vi "LV8_10a.vi"() -> ()   [LabVIEW 2016]
uses:
  <vilib>/imath/engines/lvmath2/RunTimeEngine/RangeToken/NIMS_Range.vi
  <instcachedir>/0/NIMS_Range_A7C094595B484CA7AF10685B02D808ED.lvgen/NIMS_Range_A7C094595B484CA7AF10685B02D808ED_000.vi
  <vilib>/imathl/engines/lvmath/Functions/Error Handling/Create Error.vi
  <vilib>/imath/engines/lvmath2/RunTimeEngine/BuiltInFunctions/abs/NIMS_abs(signed).vi
  <instcachedir>/0/NIMS_abs(signed)_C4FCB8E6058B49B797C7C8D53CA5F6EC.lvgen/NIMS_abs(signed)_C4FCB8E6058B49B797C7C8D53CA5F6EC_001.vi
  <vilib>/imath/engines/lvmath2/RunTimeEngine/BuiltInFunctions/fft/NIMS_fft(GV).vi
  <instcachedir>/0/NIMS_fft(GV)_4C6467FC22F84E4BA42517A07EF978B0.lvgen/NIMS_fft(GV)_4C6467FC22F84E4BA42517A07EF978B0_000.vi
  <instcachedir>/0/NIMS_abs(signed)_C4FCB8E6058B49B797C7C8D53CA5F6EC.lvgen/NIMS_abs(signed)_C4FCB8E6058B49B797C7C8D53CA5F6EC_006.vi
  <vilib>/imath/engines/lvmath2/RunTimeEngine/BuiltInFunctions/fftshift/NIMS_fftshift(GV).vi
  <instcachedir>/0/NIMS_fftshift(GV)_BD7A7BA9CA6B470B9A9F73A6A3FEEB3E.lvgen/NIMS_fftshift(GV)_BD7A7BA9CA6B470B9A9F73A6A3FEEB3E_001.vi
  <vilib>/imath/engines/lvmath2/RunTimeEngine/ErrorHandling/NIMS_Error From Error Code.vi
  <vilib>/imath/engines/lvmath2/RunTimeEngine/IndexRead/NIMS V(S).vi
  <instcachedir>/0/NIMS V(S)_0488751826AF41519A22953C041130DC.lvgen/NIMS V(S)_0488751826AF41519A22953C041130DC_000.vi
  <vilib>/imath/engines/lvmath2/RunTimeEngine/BuiltInFunctions/linramp/NIMS_linramp.vi
  <vilib>/imath/engines/lvmath2/RunTimeEngine/ErrorHandling/NIMS_Create Error From Enums.vi
  <vilib>/imath/engines/lvmath2/RunTimeEngine/ArithmeticOperatorToken/NIMS_ArithmeticOperator_times.vi
  <instcachedir>/0/NIMS_ArithmeticOperator_times_953B34F74CAC448FB707D816A29CC5F0.lvgen/NIMS_ArithmeticOperator_times_953B34F74CAC448FB707D816A29CC5F0_000.vi
  <vilib>/imath/engines/lvmath2/RunTimeEngine/NodeEndStatement/NIMS_NodeEndStatement_Output.vi
  <instcachedir>/0/NIMS_NodeEndStatement_Output_53EC0D466D134D7ABD903AC30B43404B.lvgen/NIMS_NodeEndStatement_Output_53EC0D466D134D7ABD903AC30B43404B_005.vi
  <vilib>/imath/engines/lvmath2/RunTimeEngine/ErrorHandling/NIMS_Finalize Error.vi
panel:
  in  "stop":bool
  in  "Fmax":dbl(slide)=1.5 scale=0.5..8.0
  in  "Tmax":dbl(slide)=8.0 scale=5.0..10.0
  out "Time Domain":cluster{"f":dbl[], "FX":dbl[]}[](graph)=[{"f"=[-8.0, -7.666666666666667, -7.333333333333333, -7.0, -6.666666666666667, -6.333333333333334, -6.0, -5.666666666666667, -5.333333333333334, -5.0, -4.666666666666667, -4.333333333333334, -4.0, -3.666666666666667, -3.333333333333334, -3.0, -2.666666666666667, -2.333333333333334, -2.0, -1.666666666666667, -1.333333333333334, -1.0, -0.666666666666667, -0.3333333333333339, 0.0, 0.33333333333333215, 0.6666666666666661, 1.0, 1.3333333333333321, 1.666666666666666, 2.0, 2.333333333333332, 2.666666666666666, 3.0, 3.333333333333332, 3.666666666666666, 4.0, 4.333333333333332, 4.666666666666666, 5.0, 5.333333333333332, 5.666666666666666, 6.0, 6.333333333333332, 6.666666666666666, 7.0, 7.333333333333332, 7.666666666666666], "FX"=[0.00033546262790251185, 0.00046817581165277687, 0.0006533919798673806, 0.0009118819655545162, 0.0012726338013398079, 0.0017761035457343776, 0.0024787521766663585, 0.0034593773364647584, 0.004827949993831437, 0.006737946999085467, 0.009403562551495206, 0.013123728736940956, 0.01831563888873418, 0.025561533206507392, 0.035673993347252374, 0.049787068367863944, 0.06948345122280151, 0.09697196786440501, 0.1353352832366127, 0.18887560283756177, 0.2635971381157266, 0.36787944117144233, 0.5134171190325919, 0.7165313105737888, 1.0, 0.71653131057379, 0.5134171190325924, 0.36787944117144233, 0.2635971381157271, 0.18887560283756194, 0.1353352832366127, 0.09697196786440518, 0.06948345122280157, 0.049787068367863944, 0.03567399334725244, 0.025561533206507413, 0.01831563888873418, 0.013123728736940978, 0.009403562551495213, 0.006737946999085467, 0.004827949993831446, 0.0034593773364647615, 0.0024787521766663585, 0.0017761035457343807, 0.001272633801339809, 0.0009118819655545162, 0.0006533919798673813, 0.0004681758116527773]}, {"f"=array[2000 elements], "FX"=array[2000 elements]}]
  out "Frequency Domain":cluster{"f":dbl[], "FX":dbl[]}[](graph)=[{"f"=[-1.5, -1.4375, -1.375, -1.3125, -1.25, -1.1875, -1.125, -1.0625, -1.0, -0.9375, -0.875, -0.8125, -0.75, -0.6875, -0.625, -0.5625, -0.5, -0.4375, -0.375, -0.3125, -0.25, -0.1875, -0.125, -0.0625, 0.0, 0.0625, 0.125, 0.1875, 0.25, 0.3125, 0.375, 0.4375, 0.5, 0.5625, 0.625, 0.6875, 0.75, 0.8125, 0.875, 0.9375, 1.0, 1.0625, 1.125, 1.1875, 1.25, 1.3125, 1.375, 1.4375], "FX"=[0.02226515944178319, 0.02421939412982579, 0.026441426858600965, 0.0289822550063039, 0.0319055455432762, 0.035291582471107676, 0.039242715825752186, 0.043890996174620715, 0.04940904606371528, 0.056025817636194575, 0.06404988004138219, 0.07390457496707327, 0.08618234237602979, 0.1017308444117388, 0.1217933569285751, 0.14824458322471679, 0.18399933670075047, 0.2337427294890504, 0.30526649687916235, 0.4119197872099028, 0.576800878284002, 0.837551410127783, 1.2369729163176726, 1.732783071437599, 2.0, 1.732783071437599, 1.2369729163176726, 0.837551410127783, 0.576800878284002, 0.4119197872099028, 0.30526649687916235, 0.2337427294890504, 0.18399933670075047, 0.14824458322471679, 0.1217933569285751, 0.1017308444117388, 0.08618234237602979, 0.07390457496707327, 0.06404988004138219, 0.056025817636194575, 0.04940904606371528, 0.043890996174620715, 0.039242715825752186, 0.035291582471107676, 0.0319055455432762, 0.0289822550063039, 0.026441426858600965, 0.02421939412982579]}, {"f"=array[2000 elements], "FX"=array[2000 elements]}]
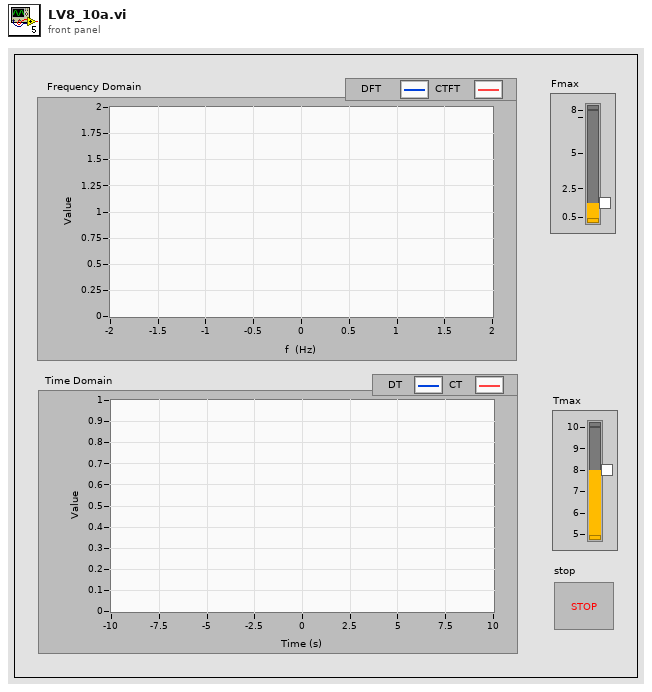
[diagram p1: front panel]
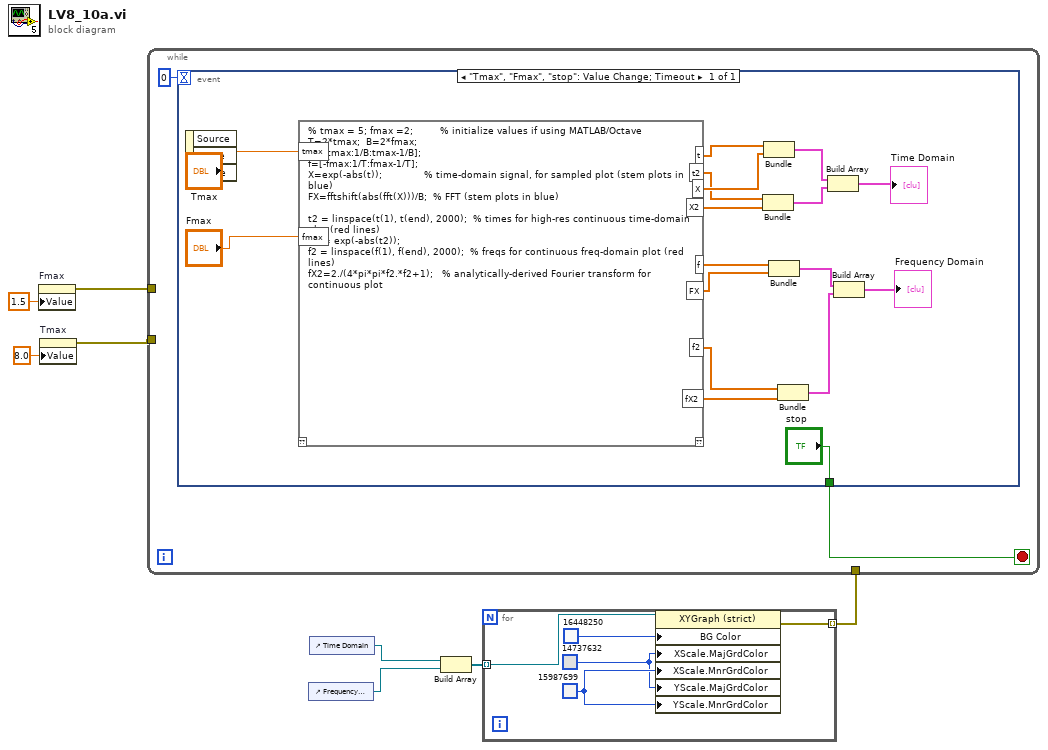
[diagram p0: block diagram]
diagram:
  n1 = property on="Fmax" class="Slide (strict)"("Value"=1.5 ("Fmax")) -> (error out=w6:errorcluster)  [unwired: 2 in, 1 out]
  n2 = property on="Tmax" class="Slide (strict)"("Value"=8.0 ("Tmax")) -> (error out=w5:errorcluster)  [unwired: 2 in, 1 out]
  n3 = control-ref of="Frequency Domain"() -> (w2:refnum<vi>)
  n4 = control-ref of="Time Domain"() -> (w3:refnum<vi>)
  n5 = Build Array(w3, w2) -> (w4:refnum<vi>[])
  n6 = for {
    tunnel: w4 -> [w10] mode=indexing
    tunnel: [w9] -> w1 mode=indexing
    w12 = u32 15987699
    w11 = u32 14737632
    n7 = property class="XYGraph (strict)"(reference=w10, "BG Color"=u32 16448250, "XScale.MajGrdColor"=w11, "XScale.MnrGrdColor"=w12, "YScale.MajGrdColor"=w11, "YScale.MnrGrdColor"=w12) -> (error out=w9:errorcluster)  [unwired: 1 in, 1 out]
  }
  n8 = while {
    tunnel: w6 -> [_]
    tunnel: w5 -> [_]
    tunnel: w1 -> [_]
    stop <- w15 stop-if-true
    n9 = event shown="[0] \"Tmax\", \"Fmax\", \"stop\": Value Change;  Timeout" {
      selector: _ -> [_]
      dyn-events: _ -> [_]
      timeout: 0 -> [_]
      tunnel: ["stop"] -> w15
      event "Tmax", "Fmax", "stop": Value Change; Timeout {
        n10 = event-data() -> ()  [unwired: 1 in, 3 out]
        n11 = mathscript code="% tmax = 5; fmax =2;         % initialize values if using MATLAB/Octave\nT=2*tmax;  B=2*fmax;\nt=[-tmax:1/B:tmax-1/B];\nf=[-fmax:1/T:fmax-1/T];\nX=exp(-abs(t));              % time-domain signal, for sampled plot (stem plots in blue)\nFX=fftshift(abs(fft(X)))/B;  % FFT (stem plots in blue)\n\nt2 = linspace(t(1), t(end), 2000);  % times for high-res continuous time-domain plot (red lines)\nX2 = exp(-abs(t2));\nf2 = linspace(f(1), f(end), 2000);  % freqs for continuous freq-domain plot (red lines)\nfX2=2./(4*pi*pi*f2.*f2+1);   % analytically-derived Fourier transform for continuous plot"("tmax"="Tmax", "fmax"="Fmax") -> ("f"=w31:dbl[], "FX"=w32:dbl[], "fX2"=w26:dbl[], "f2"=w27:dbl[], "t"=w25:dbl[], "t2"=w23:dbl[], "X"=w24:dbl[], "X2"=w22:dbl[])  [unwired: 1 in, 1 out]
        n12 = Bundle("t2"=w23, "X2"=w22) -> (w20:cluster{"t2":dbl[], "X2":dbl[]})  [unwired: 1 in]
        n13 = Bundle("t"=w25, "X"=w24) -> (w21:cluster{"t":dbl[], "X":dbl[]})  [unwired: 1 in]
        n14 = Bundle("f"=w31, "FX"=w32) -> (w30:cluster{"f":dbl[], "FX":dbl[]})  [unwired: 1 in]
        n15 = Bundle("f2"=w27, "fX2"=w26) -> (w29:cluster{"f2":dbl[], "fX2":dbl[]})  [unwired: 1 in]
        n16 = Build Array(w21, w20) -> (→"Time Domain":cluster{"t2":dbl[], "X2":dbl[]}[])
        n17 = Build Array(w30, w29) -> (→"Frequency Domain":cluster{"f2":dbl[], "fX2":dbl[]}[])
      }
    }
  }
